vi "Get SMO Serial Number.vi"(8 "error in (no error)":errorcluster, 11 "Inst.Xeryon-Rotator in":refnum<class "Inst.Xeryon-Rotator.lvclass">) -> (0 "error out":errorcluster, 2 "Serial Number":string, 3 "Inst.Xeryon-Rotator out":refnum<class "Inst.Xeryon-Rotator.lvclass">)   [LabVIEW 2019, in "Inst.Xeryon-Rotator.lvclass"]
doc: "Override this VI to return the serial number of your Instrument"
uses:
  Inst.Xeryon-Rotator.lvclass
  <userlib>/LevyLab/Instrument Framework/Instrument Types/Cryostat/Instrument.Cryostat.lvclass
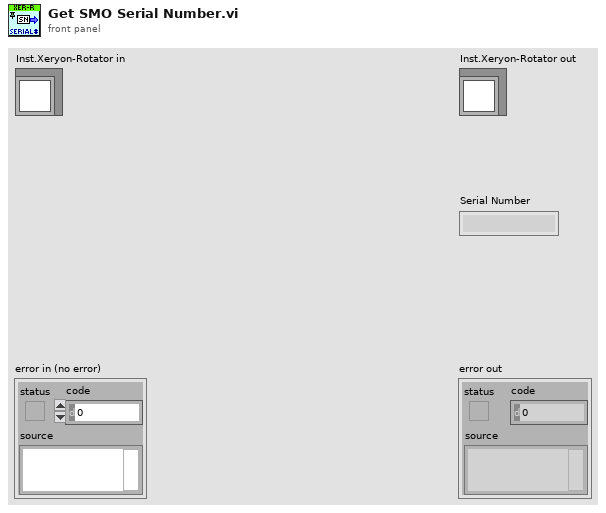
[diagram p1: front panel]
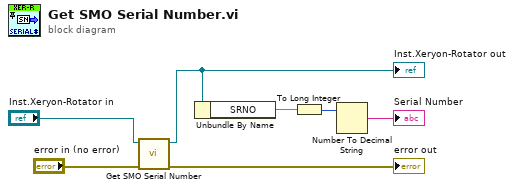
[diagram p0: block diagram]
diagram:
  n1 = call-parent "Get SMO Serial Number.vi"("error in (no error)"="error in (no error)", "Instrument in"="Inst.Xeryon-Rotator in") -> ("error out"=→"error out":errorcluster, "Instrument out"=w4:refnum<class "Inst.Xeryon-Rotator.lvclass">)  [unwired: 7 in, 1 out]
  "Inst.Xeryon-Rotator out" <- w4
  n2 = Unbundle By Name(w4) -> ("SRNO"=w3:dbl)
  n3 = To Long Integer(number=w3) -> (32bit integer=w2:i32)
  n4 = Number To Decimal String(number=w2) -> (decimal integer string=→"Serial Number":string)  [unwired: 1 in]
